vi "Read State.vi"(8 "error in (no error)":errorcluster, 11 "Change Filter State in":refnum<class "Change Filter State.lvclass">) -> (0 "error out":errorcluster, 2 "State":bool, 3 "Change Filter State out":refnum<class "Change Filter State.lvclass">)   [LabVIEW 2014, in "Controller.lvlib" / "Change Filter State.lvclass"]
uses:
  Change Filter State.lvclass
  Change Filter State.lvclass/Change Filter State.ctl
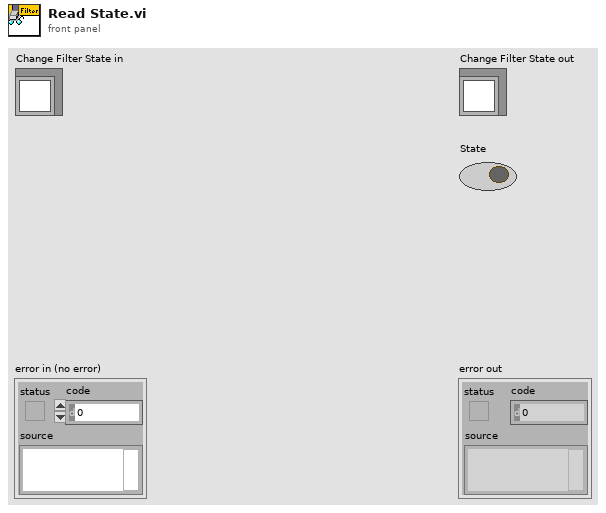
[diagram p1: front panel]
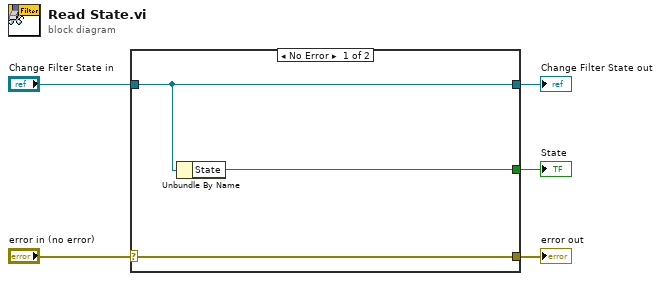
[diagram p0: block diagram]
diagram:
  n1 = case shown="No Error" "error in (no error)" {
    selector: "error in (no error)" -> [w8 w9]
    tunnel: [w8 w9] -> w4
    tunnel: [w7 w10] -> w2
    tunnel: "Change Filter State in" -> [w7 w10]
    tunnel: [w6 _] -> w1
    frame No Error {
      n2 = Unbundle By Name(w7) -> ("State"=w6:bool)
    }
    frame Error {
    }
  }
  "error out" <- w4
  "Change Filter State out" <- w2
  "State" <- w1
